vi "Write IDN.vi"(8 "error in (no error)":errorcluster, 11 "Instrument in":refnum<class "Instrument.lvclass">) -> (0 "error out":errorcluster, 3 "Instrument out":refnum<class "Instrument.lvclass">)   [LabVIEW 2019, in "Instrument.lvclass"]
doc: "Sets the <b>IDN</b> data field:\n- <b>vendor</b> is set by overriding <b>Get SMO Vendor.vi</b>\n- <b>model</b> is set by overriding <b>Get SMO Name.vi</b>\n- <b>serial</b> is set by overriding <b>Get SMO Serial Number.vi</b>\n- <b>firmware</b> refers to the version of your application"
uses:
  Instrument.lvclass
  Typedefs/Instrument.IDN--cluster.ctl
  Typedefs/Instrument.ProtectedCommands--Enum.ctl
  <vilib>/Utility/Data Type/Get Numeric Information.vi
  API/Instrument.sendMessageToProcess (variant).vi
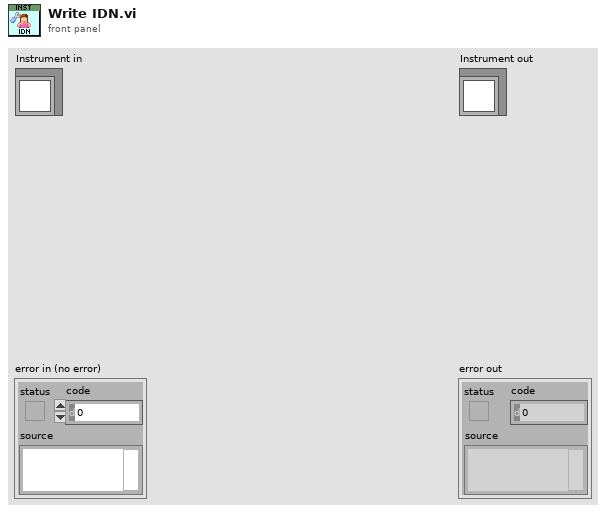
[diagram p1: front panel]
types:
  T1 = typedef "Instrument.lvclass/Instrument.ProtectedCommands--Enum.ctl" = enum16{"setConfiguration", "setLogData", "setIDN", "setAll", "setAllData"}
  T2 = typedef "Instrument.lvclass/Instrument.IDN--cluster.ctl" = cluster{"vendor":string, "model":string, "serial":string, "firmware":string}
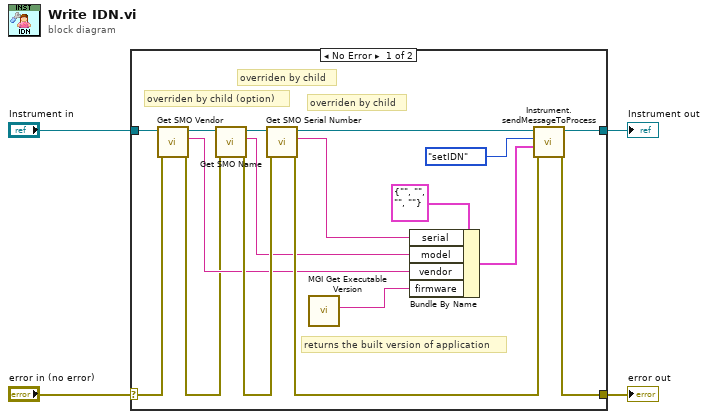
[diagram p0: block diagram]
diagram:
  n1 = case shown="No Error" "error in (no error)" {
    selector: "error in (no error)" -> [w8 w23]
    tunnel: [w16 w23] -> w3
    tunnel: [w14 w22] -> w1
    tunnel: "Instrument in" -> [w11 w22]
    frame No Error {
      # "overriden by child (option)"
      # "returns the built version of application"
      # "overriden by child"
      # "overriden by child"
      n2 = call-dynamic "Get SMO Vendor.vi"("error in (no error)"=w8, "Instrument in"=w11) -> ("error out"=w7:errorcluster, "SMO Vendor"=w9:string, "Instrument out"=w10:refnum<class "Instrument.lvclass">)  [unwired: 7 in]
      n3 = call-dynamic "Get SMO Name.vi"("error in (no error)"=w7, "Instrument in"=w10) -> ("error out"=w20:errorcluster, "SMO Name"=w12:string, "Instrument out"=w6:refnum<class "Instrument.lvclass">)  [unwired: 7 in]
      n4 = call-dynamic "Get SMO Serial Number.vi"("error in (no error)"=w20, "Instrument in"=w6) -> ("error out"=w17:errorcluster, "Serial Number"=w13:string, "Instrument out"=w15:refnum<class "Instrument.lvclass">)  [unwired: 7 in]
      n5 = call <userlib>:"MGI Get Executable Version.vi"() -> ("Version"=w21:string)  [unwired: 7 in]
      n6 = Bundle By Name(cluster=T2 {"vendor"="", "model"="", "serial"="", "firmware"=""} ("IDN"), "serial"=w13, "model"=w12, "vendor"=w9, "firmware"=w21) -> (w18:T2)
      n7 = call-poly "Instrument.sendMessageToProcess.vi"("error in (no error)"=w17, "Data"=w18, "Command"=Instrument.ProtectedCommands--Enum."setIDN" ("PrivateCommands"), "Instrument"=w15) -> ("error out"=w16:errorcluster, "Instrument out"=w14:refnum<class "Instrument.lvclass">)  [unwired: 6 in]
    }
    frame Error {
    }
  }
  "error out" <- w3
  "Instrument out" <- w1
